vi "Read lockin time constant.vi"(8 "error in (no error)":errorcluster, 11 "Lockin SR830.lvclass In":refnum<class "Lockin SR830.lvclass">) -> (0 "error out":errorcluster, 2 "Tau":u16(ring) items=["10 us", "30 us", "100 us", "300 us", "1 ms", "3 ms", "10 ms", "30 ms", "100 ms", "300 ms", "1 s", "3 s", "10 s", "30 s", "100 s", "300 s", "1 ks", "3 ks", "10 ks", "30 ks"], 3 "Lockin SR830.lvclass out":refnum<class "Lockin SR830.lvclass">)   [LabVIEW 2017, in "Lockin SR830.lvclass"]
doc: "Reads the current time constant from the lock-in detector."
uses:
  Lockin SR830.lvclass
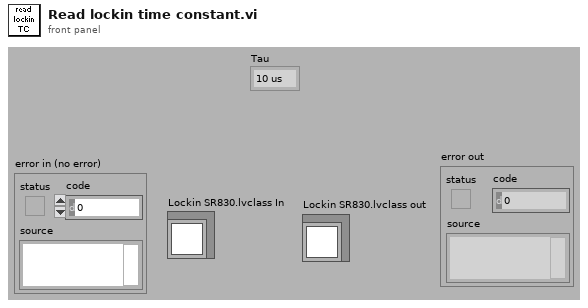
[diagram p1: front panel]
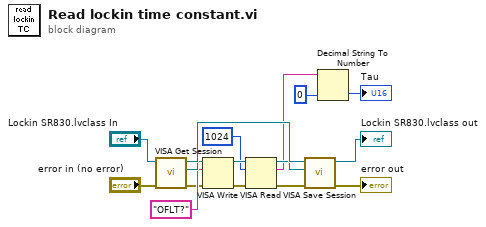
[diagram p0: block diagram]
diagram:
  n1 = call-dynamic "VISA Get Session.vi"("error in (no error)"="error in (no error)", "Instrument.lvclass in"="Lockin SR830.lvclass In") -> ("error out"=w5:errorcluster, "VISA Resource Name"=w7:refnum<visa-resource-name>, "Instrument.lvclass out"=w14:refnum<class "Lockin SR830.lvclass">)  [unwired: 6 in, 1 out]
  n2 = VISA Write(VISA resource name=w7, write buffer="OFLT?" ("data"), error in (no error)=w5) -> (VISA resource name out=w8:refnum<visa-resource-name>, error out=w9:errorcluster)  [unwired: 1 out]
  n3 = VISA Read(VISA resource name=w8, byte count=u32 1024, error in (no error)=w9) -> (VISA resource name out=w3:refnum<visa-resource-name>, read buffer=w2:string, error out=w4:errorcluster)  [unwired: 1 out]
  n4 = call-dynamic "VISA Save Session.vi"("error in (no error)"=w4, "VISA Resource Name"=w3, "Instrument.lvclass in"=w14) -> ("error out"=→"error out":errorcluster, "Instrument.lvclass out"=→"Lockin SR830.lvclass out":refnum<class "Lockin SR830.lvclass">)  [unwired: 7 in]
  n5 = Decimal String To Number(string=w2, default (0L)=u16 0 ("default (0 I32)")) -> (number=→"Tau":u16)  [unwired: 2 out]
